vi "Search DB for Item Data.vi"(4 "Measurement? (F)":bool, 6 "Windows? (F)":bool, 8 "error in (no error)":errorcluster, 9 "Item Name":string, 10 "DB Path":path, 11 "Custom Device Node in":refnum<k24>) -> (0 "error out":errorcluster, 1 "Comment":string, 2 "Extension":u8, 3 "Address":u32 format="%x", 5 "Unit":string)   [LabVIEW 2011]
uses:
  NationalInstruments.VeriStand.SystemStorage
  <vilib>/ECUMC/ECUMC.llb/MC Get Prop Meas Comment.vi
  <vilib>/ECUMC/ECUMC.llb/MC Get Prop Meas Extension.vi
  <vilib>/ECUMC/ECUMC.llb/MC Get Prop Meas Address.vi
  <vilib>/ECUMC/ECUMC.llb/MC Get Prop Meas Unit.vi
  <vilib>/ECUMC/ECUMC.llb/MC Get Prop Char Comment.vi
  <vilib>/ECUMC/ECUMC.llb/MC Get Prop Char Extension.vi
  <vilib>/ECUMC/ECUMC.llb/MC Get Prop Char Address.vi
  <vilib>/ECUMC/ECUMC.llb/MC Get Prop Char Unit.vi
  <vilib>/ECUMC/ECUMC.lvlib
panel:
  in  "ECU name":string
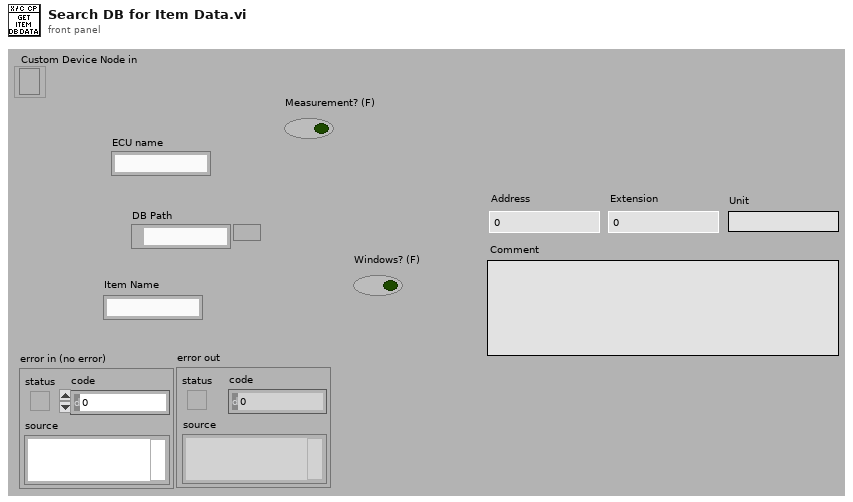
[diagram p1: front panel]
types:
  T1 = typedef "ECUMC.lvlib/MC Reference.ctt" = u32
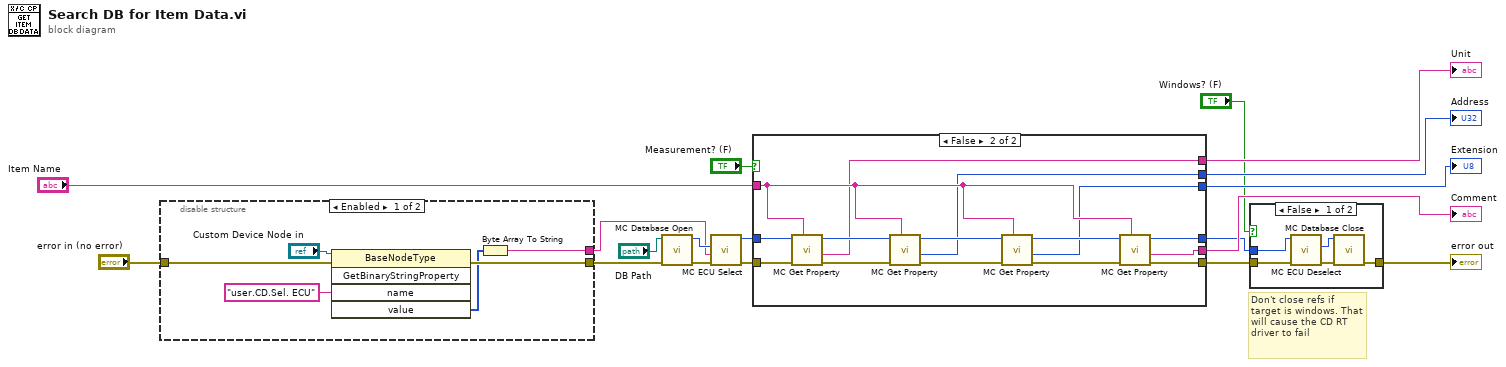
[diagram p0: block diagram]
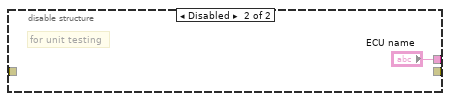
[diagram p2: hidden frame]
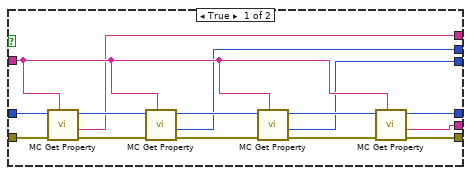
[diagram p4: hidden frame]
diagram:
  # "Don't close refs if target is windows. That will cause the CD RT driver to fail"
  n1 = disable-structure shown="Enabled" {
    disable-tunnel: [w23 _] -> w10
    disable-tunnel: [w20 "ECU name"] -> w7
    disable-tunnel: "error in (no error)" -> [w19 _]
    frame Enabled {
      n2 = invoke class="BaseNodeType" method="GetBinaryStringProperty"(reference="Custom Device Node in", error in=w19, "name"="user.CD.Sel. ECU") -> (error out=w23:errorcluster, "value"=w21:u8[])  [unwired: 2 in, 3 out]
      n3 = Byte Array To String(unsigned byte array=w21) -> (string=w20:string)
    }
    frame Disabled {
      # "for unit testing"
    }
  }
  n4 = call <vilib>:"MC Database Open.vi"("error in"=w10, "DB path"="DB Path") -> ("error out"=w9:errorcluster, "DB ref out"=w8:T1)  [unwired: 8 in]
  n5 = call <vilib>:"MC ECU Select.vi"("error in"=w9, "ECU name"=w7, "DB ref in"=w8) -> ("error out"=w3:errorcluster, "ECU ref out"=w2:T1)  [unwired: 7 in]
  n6 = case shown="False" "Measurement? (F)" {
    tunnel: [w33 w48] -> w5
    tunnel: w3 -> [w40 w55]
    tunnel: w2 -> [w39 w54]
    tunnel: "Item Name" -> [w38 w53]
    tunnel: [w34 w49] -> w1
    tunnel: [w29 w44] -> w17
    tunnel: [w28 w43] -> w16
    tunnel: [w27 w42] -> w15
    tunnel: [w26 w41] -> w14
    frame True {
      n7 = call-poly <vilib>:"MC Get Property.vi"("name"=w38, "error in"=w40, "reference in"=w39) -> ("error out"=w30:errorcluster, "unit"=w29:string, "reference out"=w37:T1)  [unwired: 6 in]
      n8 = call-poly <vilib>:"MC Get Property.vi"("name"=w38, "error in"=w30, "reference in"=w37) -> ("error out"=w31:errorcluster, "meas address"=w28:u32, "reference out"=w36:T1)  [unwired: 6 in]
      n9 = call-poly <vilib>:"MC Get Property.vi"("name"=w38, "error in"=w31, "reference in"=w36) -> ("error out"=w32:errorcluster, "meas extension"=w27:u8, "reference out"=w35:T1)  [unwired: 6 in]
      n10 = call-poly <vilib>:"MC Get Property.vi"("name"=w38, "error in"=w32, "reference in"=w35) -> ("error out"=w33:errorcluster, "comment"=w26:string, "reference out"=w34:T1)  [unwired: 6 in]
    }
    frame False {
      n11 = call-poly <vilib>:"MC Get Property.vi"("name"=w53, "error in"=w55, "reference in"=w54) -> ("error out"=w45:errorcluster, "unit"=w44:string, "reference out"=w52:T1)  [unwired: 6 in]
      n12 = call-poly <vilib>:"MC Get Property.vi"("name"=w53, "error in"=w45, "reference in"=w52) -> ("error out"=w46:errorcluster, "char address"=w43:u32, "reference out"=w51:T1)  [unwired: 6 in]
      n13 = call-poly <vilib>:"MC Get Property.vi"("name"=w53, "error in"=w46, "reference in"=w51) -> ("error out"=w47:errorcluster, "char extension"=w42:u8, "reference out"=w50:T1)  [unwired: 6 in]
      n14 = call-poly <vilib>:"MC Get Property.vi"("name"=w53, "error in"=w47, "reference in"=w50) -> ("error out"=w48:errorcluster, "comment"=w41:string, "reference out"=w49:T1)  [unwired: 6 in]
    }
  }
  "Address" <- w16
  "Extension" <- w15
  "Unit" <- w17
  "Comment" <- w14
  n15 = case shown="False" "Windows? (F)" {
    tunnel: w5 -> [w60 w61]
    tunnel: [w57 w61] -> w18
    tunnel: w1 -> [w56 _]
    frame False {
      n16 = call <vilib>:"MC ECU Deselect.vi"("error in"=w60, "ECU ref in"=w56) -> ("error out"=w59:errorcluster, "DB ref out"=w58:T1)  [unwired: 8 in]
      n17 = call <vilib>:"MC Database Close.vi"("error in"=w59, "DB ref in"=w58) -> ("error out"=w57:errorcluster)  [unwired: 9 in]
    }
    frame True {
    }
  }
  "error out" <- w18
